vi "Strip Path Extension - Path__ogtk.vi"(0 "path":path) -> (1 "root":string, 2 "extension":string)   [LabVIEW 2011]
panel:
  # "[OpenG VI Tags] ***Do Not Remove***\nCVS Revision = 1.2\nCVS Revision Date = Thu Nov  6 19:59:27 2003\nPackage = oglib_file-2.2-1\nDepends ="
  # "Strip Path Extension.vi - Splits a relative or absolute path\ninto its root and extension.  Path can be a string or a path.\n\nCopyright (C) 2002 James Kring jim@jimkring.com\n\nPlease visit http://www.OpenG.org to learn about the\nOpen Source LabVIEW software movement.\n\nThis library is free software; you can redistribute it and/or\nmodify it under the terms of the GNU Lesser General Public\nLicense as published by the Free Software Foundation; either\nversion 2.1 of the License, or (at your option) any later version.\nThis library is distributed in the hope that it will be useful,\nbut WITHOUT ANY WARRANTY; without even the implied warranty of\nMERCHANTABILITY or FITNESS FOR A PARTICULAR PURPOSE. See the GNU\nLesser General Public License for more details.\nYou should have received a copy of the GNU Lesser General Public\nLicense along with this library; if not, write to the Free Software\nFoundation, Inc., 59 Temple Place, Suite 330, Boston, MA 02111-1307 USA"
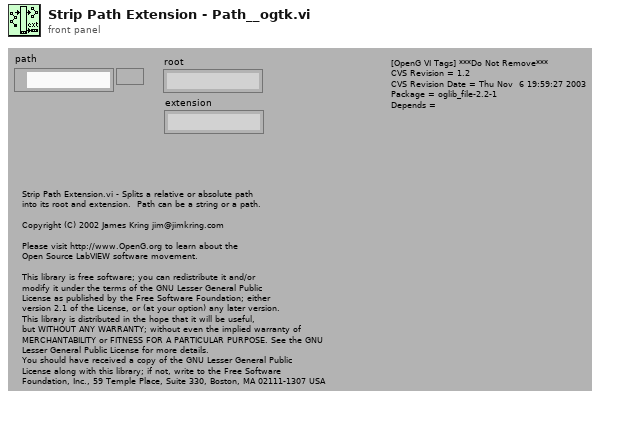
[diagram p1: front panel]
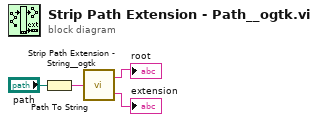
[diagram p0: block diagram]
diagram:
  n1 = Path To String(path="path") -> (string=w3:string)
  n2 = call "Strip Path Extension - String__ogtk.vi"("path"=w3) -> ("root"=→"root":string, "extension"=→"extension":string)
